vi "_PC_Pub_Freq2Decyc.vi"(8 "Freq":ext) -> (0 "(1/Decyc)*2^8":u32, 1 "Decyc*2^32":u32, 2 "1/Decyc":dbl, 3 "Decyc":dbl, 4 "Actual Freq":dbl)   [LabVIEW 2018]
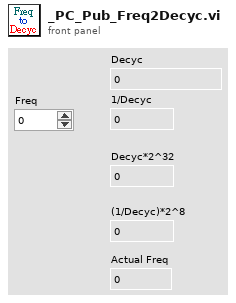
[diagram p1: front panel]
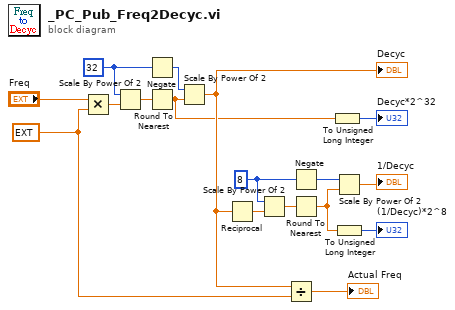
[diagram p0: block diagram]
diagram:
  w16 = i16 8 ("n")
  w13 = i16 32 ("n")
  w6 = ext 2.5e-08
  n1 = Multiply(x="Freq", y=w6) -> (x*y=w9:ext)
  n2 = Scale By Power Of 2(n=w13, x=w9) -> (x*2^n=w10:ext)
  n3 = Negate(x=w13) -> (-x=w14:i16)
  n4 = Round To Nearest(number=w10) -> (nearest integer value=w4:ext)
  n5 = Scale By Power Of 2(n=w14, x=w4) -> (x*2^n=w7:ext)
  "Decyc" <- w7
  n6 = Reciprocal(x=w7) -> (1/x=w11:ext)
  n7 = Scale By Power Of 2(n=w16, x=w11) -> (x*2^n=w12:ext)
  n8 = Divide(x=w7, y=w6) -> (x/y=→"Actual Freq":ext)
  n9 = Negate(x=w16) -> (-x=w15:i16)
  n10 = Round To Nearest(number=w12) -> (nearest integer value=w3:ext)
  n11 = To Unsigned Long Integer(number=w4) -> (unsigned 32bit integer=→"Decyc*2^32":u32)
  n12 = Scale By Power Of 2(n=w15, x=w3) -> (x*2^n=→"1/Decyc":ext)
  n13 = To Unsigned Long Integer(number=w3) -> (unsigned 32bit integer=→"(1/Decyc)*2^8":u32)
